vi "curva  com vão desnivelado.vi"() -> ()   [LabVIEW 2020]
panel:
  out "Waveform Graph":dbl[](graph)
  out "Coordenada x":dbl
  in  "B":dbl
  in  "ps":dbl
  in  "T0s":dbl
  in  "As":dbl
  out "Fs":dbl
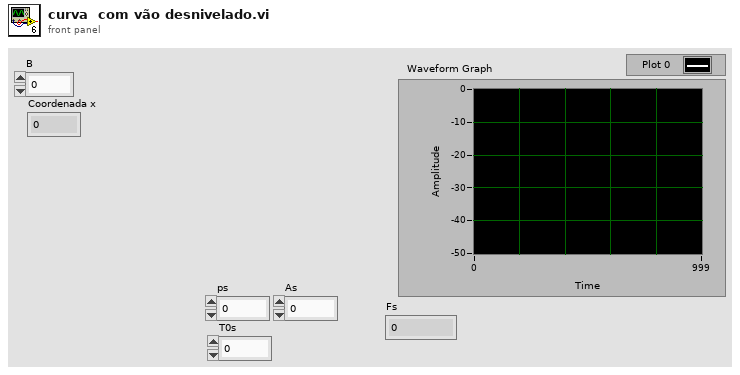
[diagram p1: front panel]
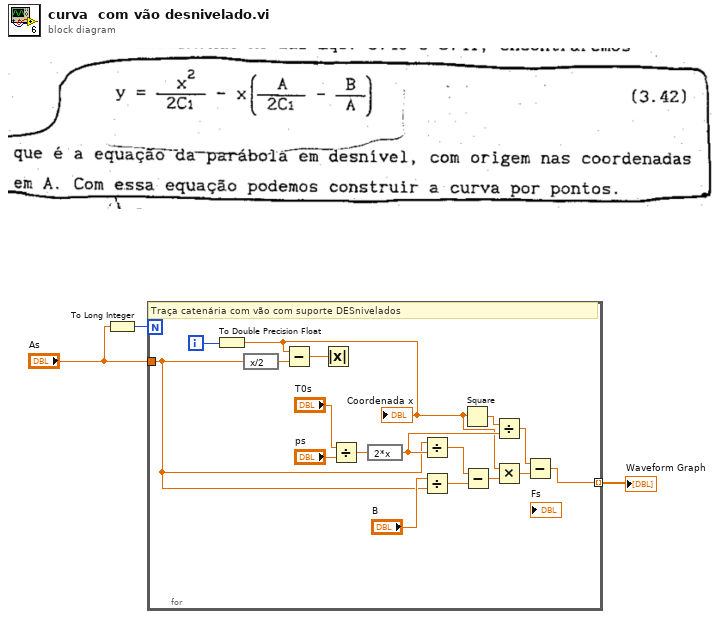
[diagram p0: block diagram]
diagram:
  n1 = To Long Integer(number="As") -> (32bit integer=w2:i32)
  n2 = for {
    N: w2 -> [_]
    tunnel: [w9] -> w3 mode=indexing
    tunnel: "As" -> [w4]
    i -> [w6]
    # "Traça catenária com vão com suporte DESnivelados"
    n3 = To Double Precision Float(number=w6) -> (double precision float=w5:dbl)
    "Coordenada x" <- w5
    n4 = expression code="x/2"(w4) -> (w8:dbl)
    n5 = Subtract(x=w5, y=w8) -> (x-y=w7:dbl)
    n6 = Absolute Value(x=w7) -> ()  [unwired: 1 out]
    n7 = Divide(x="T0s", y="ps") -> (x/y=w20:dbl)
    n8 = expression code="2*x"(w20) -> (w12:dbl)
    n9 = Divide(x=w4, y=w12) -> (x/y=w16:dbl)
    n10 = Divide(x="B", y=w4) -> (x/y=w15:dbl)
    n11 = Square(x=w5) -> (x^2=w11:dbl)
    n12 = Subtract(x=w16, y=w15) -> (x-y=w14:dbl)
    n13 = Divide(x=w11, y=w12) -> (x/y=w10:dbl)
    n14 = Multiply(x=w5, y=w14) -> (x*y=w13:dbl)
    n15 = Subtract(x=w10, y=w13) -> (x-y=w9:dbl)
  }
  "Waveform Graph" <- w3
